vi "TCP_Server+命令.vi"() -> ()   [LabVIEW 2023]
uses:
  <vilib>/measure/NI_MABase.lvlib
panel:
  in  "波形停止":bool
  in  "字符串/波形\n参数切换":enum32{"字符串", "参数"}(ring)
  out "波形图":waveform(dbl)(graph)
  out "方波占空比%":i32
  out "幅值":i32
  out "波形":i32
  out "频率":i32
  out "文件传输进度":dbl(slide) scale=0.0..100.0
  out "信息内容":string
  out "时间":string
  out "信息字节数":string
  out "文件内容":string
  out "文件字节数":string
  in  "接收文件处理（打开:0）":T1(ring)
  out "发送时间":string
  out "本机IP":string
  in  "停止":bool
  in  "接收停止":bool
  in  "停止按钮":bool
  in  "确定按钮":bool
  in  "发送字符串":string
  in  "?":bool
  in  "?":path
  in  "发送文件处理（打开:0）":T1(ring)
  in  "port":u16=7779 caption="TCP监听端口"
  # "TCP_Server"
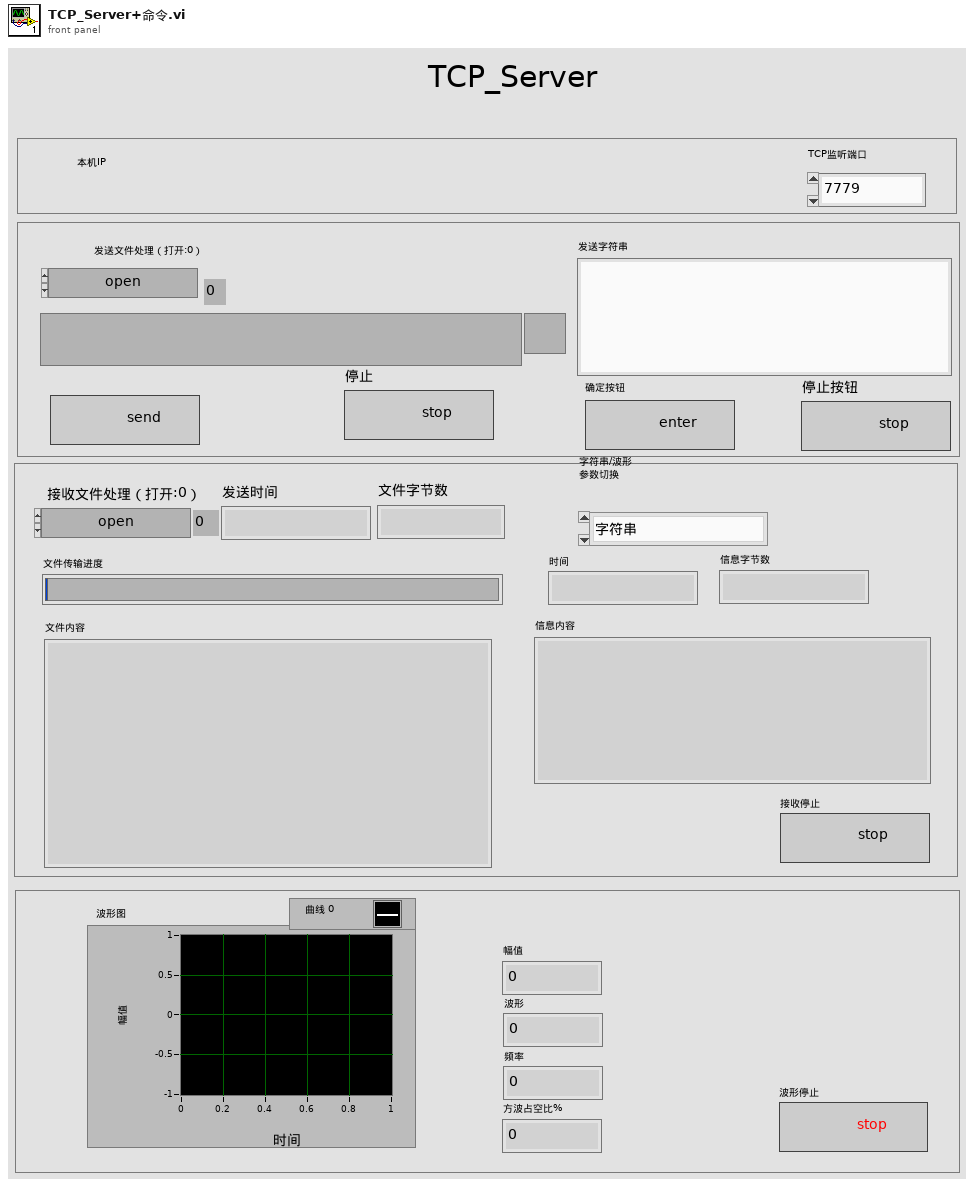
[diagram p1: front panel]
types:
  T1 = enum16{"open", "open or create", "create or replace", "create", "open (read only)"}
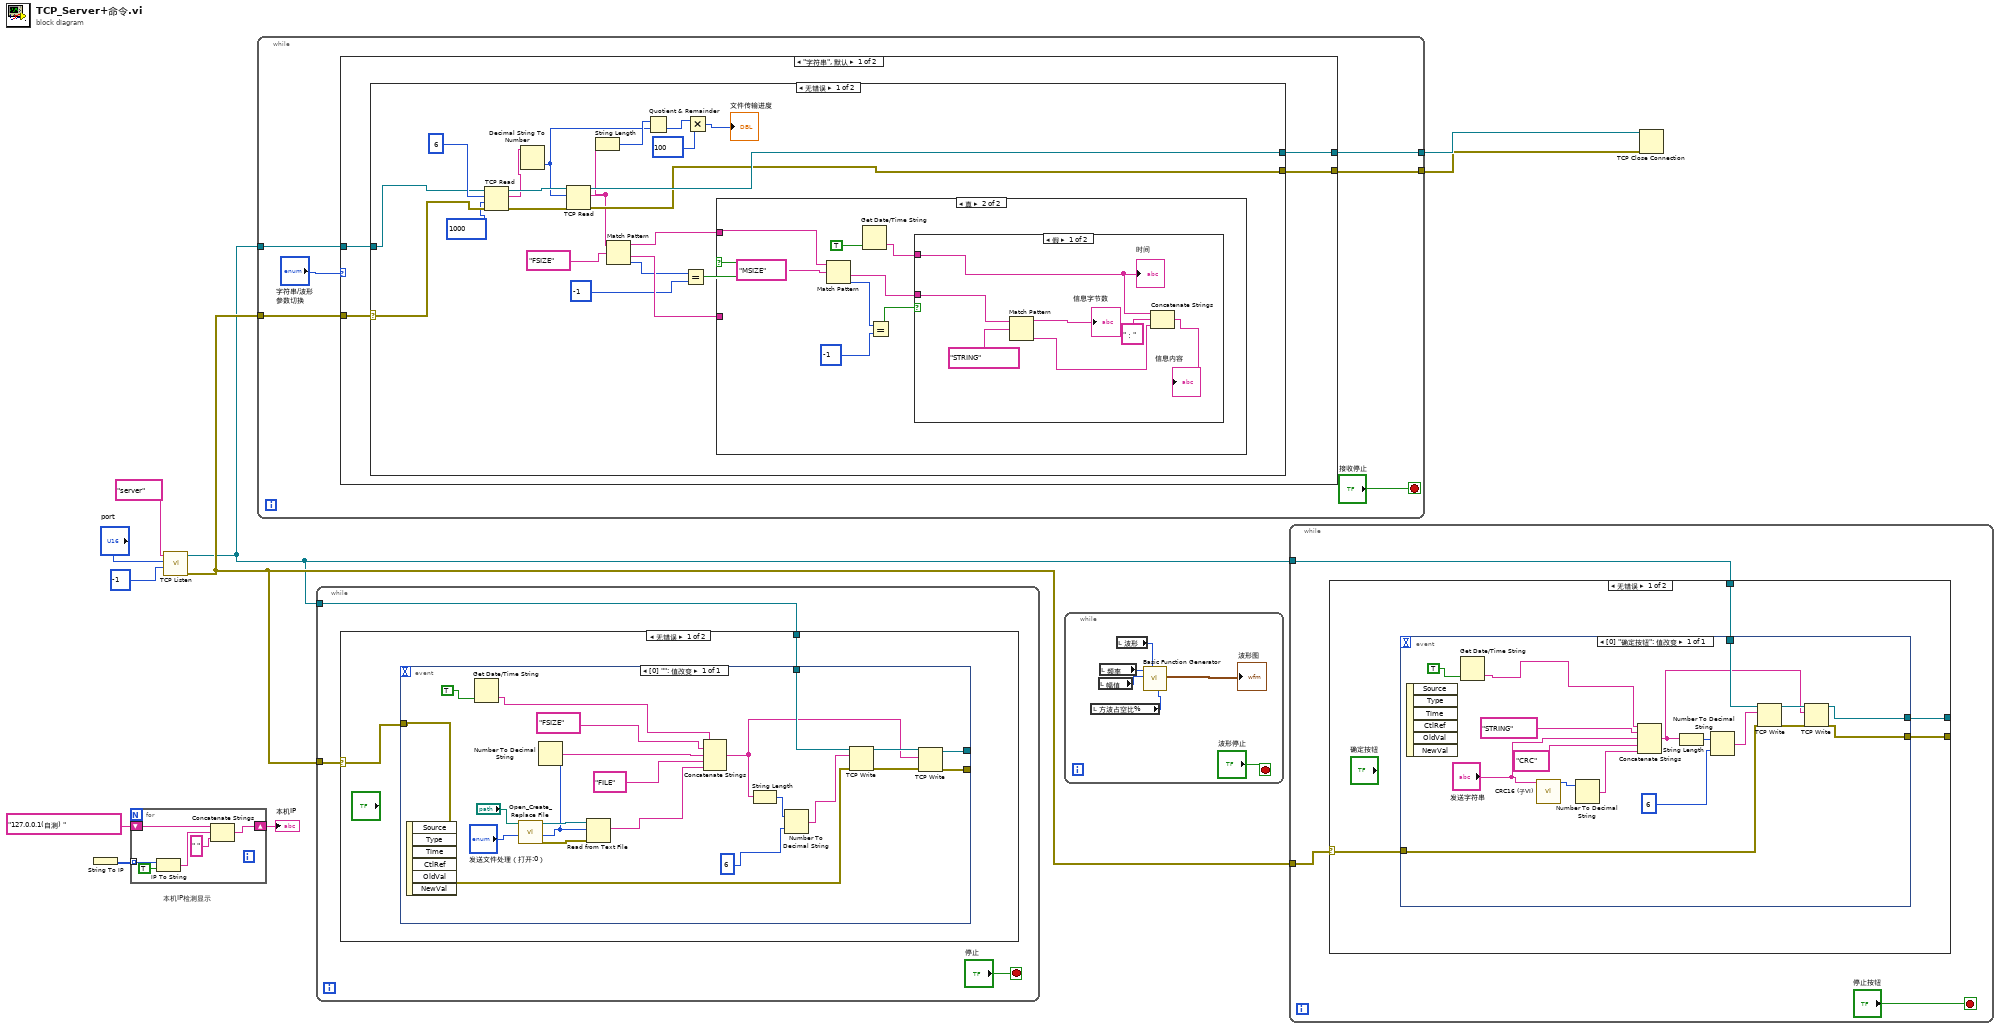
[diagram p0: block diagram]
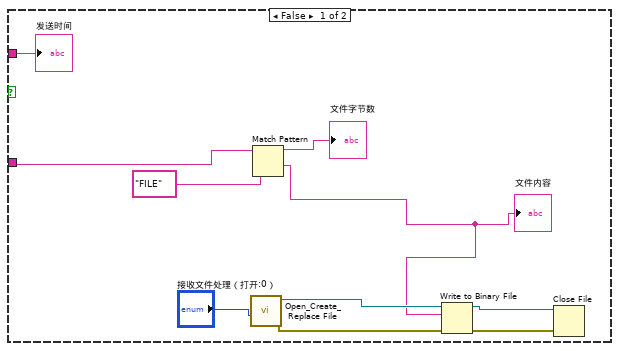
[diagram p4: hidden frame]
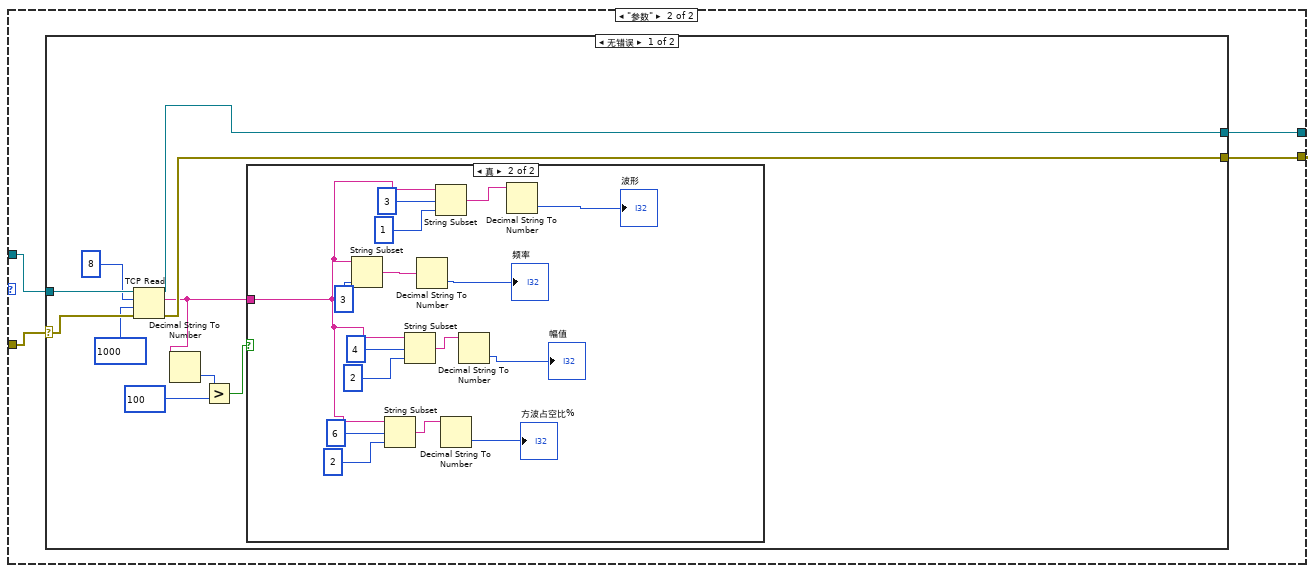
[diagram p7: hidden frame]
diagram:
  # "本机IP检测显示"
  n1 = String To IP() -> (0:w6:u32[])  [unwired: 1 in]
  n2 = for {
    tunnel: w6 -> [w16] mode=indexing
    shift-right: [w13] -> w7
    shift-left: "127.0.0.1(自测) " ("name") -> [w14]
    n3 = IP To String(1:TRUE ("句点符号？(F)"), 2:w16) -> (0:w12:string)
    n4 = Concatenate Strings(w14, w12, " " ("字符串")) -> (w13:string)
  }
  "本机IP" <- w7
  n5 = call <vilib>:"TCP Listen.vi"("timeout ms (wait forever: -1)"=-1, "port"="port", "service name"="server") -> ("error out"=w10:errorcluster, "connection ID"=w9:refnum<k5>)  [unwired: 4 in, 3 out]
  n6 = while {
    tunnel: w10 -> [w22]
    tunnel: w9 -> [w21]
    tunnel: [w19] -> w3
    tunnel: [w18] -> w2
    stop <- "接收停止" stop-if-true
    n7 = case shown="\"字符串\", 默认" "字符串/波形\n参数切换" {
      tunnel: w22 -> [w26 w75]
      tunnel: w21 -> [w25 w78]
      tunnel: [w24 w77] -> w19
      tunnel: [w23 w76] -> w18
      frame "字符串", Default {
        n8 = case shown="无错误" w26 {
          selector: w26 -> [w36 w74]
          tunnel: w25 -> [w37 w73]
          tunnel: [w35 w73] -> w24
          tunnel: [w34 w74] -> w23
          frame No Error {
            n9 = TCP Read(connection ID=w37, bytes to read=i16 6, error in (no error)=w36, 9:1000) -> (connection ID out=w41:refnum<k5>, data out=w38:string, error out=w40:errorcluster)  [unwired: 1 in]
            n10 = Decimal String To Number(string=w38) -> (number=w31:i32)  [unwired: 2 in, 1 out]
            n11 = TCP Read(connection ID=w41, bytes to read=w31, error in (no error)=w40) -> (connection ID out=w35:refnum<k5>, data out=w33:string, error out=w34:errorcluster)  [unwired: 2 in]
            n12 = String Length(string=w33) -> (length=w32:i32)
            n13 = Match Pattern(string=w33, regular expression="FSIZE") -> (before substring=w47:string, after substring=w46:string, offset past match=w44:i32)  [unwired: 1 in, 1 out]
            n14 = Quotient & Remainder(x=w32, y=w31) -> (floor(x/y)=w30:i32)  [unwired: 1 out]
            n15 = Equal?(x=w44, y=-1) -> (x = y?=w45:bool)
            n16 = Multiply(x=w30, y=100) -> (x*y=→"文件传输进度":i32)
            n17 = case shown="真" w45 {
              tunnel: w46 -> [w55 _]
              tunnel: w47 -> [w49 w64]
              frame False {
                n18 = call <vilib>:"Open_Create_Replace File.vi"("function (open:0)"="接收文件处理（打开:0）") -> ("error out"=w52:errorcluster, "refnum"=w53:refnum<file>)  [unwired: 7 in, 2 out]
                n19 = Match Pattern(string=w55, regular expression="FILE") -> (before substring=→"文件字节数":string, after substring=w48:string)  [unwired: 1 in, 2 out]
                "文件内容" <- w48
                n20 = Write to Binary File(file (use dialog)=w53, data=w48, error in=w52) -> (refnum out=w51:refnum<file>, error out=w50:errorcluster)  [unwired: 3 in, 1 out]
                n21 = Close File(refnum=w51, error in=w50) -> ()  [unwired: 2 out]
                "发送时间" <- w49
              }
              frame True {
                n22 = Match Pattern(string=w64, regular expression="MSIZE") -> (after substring=w60:string, offset past match=w63:i32)  [unwired: 1 in, 2 out]
                n23 = Get Date/Time String(want seconds? (F)=TRUE) -> (time string=w58:string)  [unwired: 2 in, 1 out]
                n24 = Equal?(x=w63, y=-1) -> (x = y?=w61:bool)
                n25 = case shown="假" w61 {
                  tunnel: w60 -> [w71 _]
                  tunnel: w58 -> [w69 _]
                  frame False {
                    n26 = Match Pattern(string=w71, regular expression="STRING") -> (before substring=→"信息字节数":string, after substring=w66:string)  [unwired: 1 in, 2 out]
                    n27 = Concatenate Strings(w69, "：", w66) -> (→"信息内容":string)
                    "时间" <- w69
                  }
                  frame True {
                  }
                }
              }
            }
          }
          frame Error {
          }
        }
      }
      frame "参数" {
        n28 = case shown="无错误" w75 {
          selector: w75 -> [w84 w105]
          tunnel: w78 -> [w88 w106]
          tunnel: [w86 w106] -> w77
          tunnel: [w85 w105] -> w76
          frame No Error {
            n29 = TCP Read(connection ID=w88, bytes to read=8, error in (no error)=w84, 9:1000) -> (connection ID out=w86:refnum<k5>, data out=w82:string, error out=w85:errorcluster)  [unwired: 1 in]
            n30 = Decimal String To Number(string=w82) -> (number=w81:i32)  [unwired: 2 in, 1 out]
            n31 = Greater?(x=w81, y=100) -> (0:w79:bool)
            n32 = case shown="真" w79 {
              tunnel: w82 -> [_ w89]
              frame False {
              }
              frame True {
                n33 = String Subset(string=w89, length (rest)=3) -> (substring=w95:string)  [unwired: 1 in]
                n34 = String Subset(string=w89, offset (0)=6, length (rest)=2) -> (substring=w96:string)
                n35 = String Subset(string=w89, offset (0)=4, length (rest)=2) -> (substring=w97:string)
                n36 = Decimal String To Number(string=w95) -> (number=→"频率":i32)  [unwired: 2 in, 1 out]
                n37 = String Subset(string=w89, offset (0)=3, length (rest)=1) -> (substring=w93:string)
                n38 = Decimal String To Number(string=w96) -> (number=→"方波占空比%":i32)  [unwired: 2 in, 1 out]
                n39 = Decimal String To Number(string=w97) -> (number=→"幅值":i32)  [unwired: 2 in, 1 out]
                n40 = Decimal String To Number(string=w93) -> (number=→"波形":i32)  [unwired: 2 in, 1 out]
              }
            }
          }
          frame Error {
          }
        }
      }
    }
  }
  n41 = while {
    tunnel: w10 -> [w109]
    tunnel: w9 -> [w108]
    stop <- "停止" stop-if-true
    n42 = case shown="无错误" w109 {
      selector: w109 -> [w111 _]
      tunnel: w108 -> [w110 _]
      frame No Error {
        n43 = event shown="[0] \"\": 值改变" {
          selector: _ -> [_]
          dyn-events: _ -> [_]
          timeout: _ -> [_]
          tunnel: w111 -> [w122]
          tunnel: w110 -> [w124]
          tunnel: [w120] -> _
          tunnel: [w119] -> _
          event Value Change {
            n44 = event-data() -> ()  [unwired: 1 in, 6 out]
            n45 = Get Date/Time String(want seconds? (F)=TRUE) -> (time string=w117:string)  [unwired: 2 in, 1 out]
            n46 = call <vilib>:"Open_Create_Replace File.vi"("function (open:0)"="发送文件处理（打开:0）", "file path"="?") -> ("error out"=w130:errorcluster, "file size (bytes)"=w128:i32, "refnum"=w129:refnum<file>)  [unwired: 6 in, 1 out]
            n47 = Number To Decimal String(number=w128) -> (decimal integer string=w126:string)  [unwired: 1 in]
            n48 = Read from Text File(file (use dialog)=w129, count=w128, error in=w130) -> (text=w112:string)  [unwired: 1 in, 3 out]
            n49 = Concatenate Strings(w117, "FSIZE", w126, "FILE", w112) -> (w113:string)
            n50 = String Length(string=w113) -> (length=w116:i32)
            n51 = Number To Decimal String(number=w116, width (-)=6) -> (decimal integer string=w114:string)
            n52 = TCP Write(connection ID=w124, data in=w114, error in (no error)=w122) -> (connection ID out=w123:refnum<k5>, error out=w121:errorcluster)  [unwired: 1 in, 1 out]
            n53 = TCP Write(connection ID=w123, data in=w113, error in (no error)=w121) -> (connection ID out=w120:refnum<k5>, error out=w119:errorcluster)  [unwired: 1 in, 1 out]
          }
        }
      }
      frame Error {
      }
    }
  }
  n54 = while {
    stop <- "波形停止" stop-if-true
    n55 = local read "方波占空比%"() -> (w138:i32)
    n56 = local read "幅值"() -> (w137:i32)
    n57 = local read "频率"() -> (w136:i32)
    n58 = local read "波形"() -> (w135:i32)
    n59 = call <vilib>:"Basic Function Generator.vi"("square wave duty cycle (%)"=w138, "signal type"=w135, "amplitude"=w137, "frequency"=w136) -> ("signal out"=→"波形图":waveform(dbl))  [unwired: 5 in, 2 out]
  }
  n60 = while {
    tunnel: w10 -> [w141]
    tunnel: w9 -> [w140]
    stop <- "停止按钮" stop-if-true
    n61 = case shown="无错误" w141 {
      selector: w141 -> [w145 w164]
      tunnel: w140 -> [w144 w163]
      tunnel: [w143 w164] -> _
      tunnel: [w142 w163] -> _
      frame No Error {
        n62 = event shown="[0] \"确定按钮\": 值改变" {
          selector: _ -> [_]
          dyn-events: _ -> [_]
          timeout: _ -> [_]
          tunnel: w145 -> [w162]
          tunnel: w144 -> [w159]
          tunnel: [w158] -> w143
          tunnel: [w157] -> w142
          event "确定按钮": Value Change {
            n63 = event-data() -> ()  [unwired: 1 in, 6 out]
            n64 = Get Date/Time String(want seconds? (F)=TRUE) -> (time string=w152:string)  [unwired: 2 in, 1 out]
            n65 = call "CRC16 (子VI).vi"("字符串"="发送字符串") -> ("数值"=w147:u16)  [unwired: 10 in]
            n66 = Number To Decimal String(number=w147) -> (decimal integer string=w146:string)  [unwired: 1 in]
            n67 = Concatenate Strings(w152, "STRING", "发送字符串", "CRC", w146) -> (w156:string)
            n68 = String Length(string=w156) -> (length=w155:i32)
            n69 = Number To Decimal String(number=w155, width (-)=6) -> (decimal integer string=w154:string)
            n70 = TCP Write(connection ID=w159, data in=w154, error in (no error)=w162) -> (connection ID out=w161:refnum<k5>, error out=w160:errorcluster)  [unwired: 1 in, 1 out]
            n71 = TCP Write(connection ID=w161, data in=w156, error in (no error)=w160) -> (connection ID out=w157:refnum<k5>, error out=w158:errorcluster)  [unwired: 1 in, 1 out]
          }
        }
      }
      frame Error {
      }
    }
  }
  n72 = TCP Close Connection(connection ID=w3, error in (no error)=w2) -> ()  [unwired: 1 in, 2 out]
